vi "aaa.vi"() -> ()   [LabVIEW 2018]
uses:
  demo/Implementations/Component-A.lvclass
  U:/modules/labview-orm/_Serializable Base Object/_ISerializable.lvclass
  demo/Implementations/Product-A.lvclass
  ORM Scripter/ORM Scripter.lvclass
panel:
  out "create script 3":string
  out "create script":string
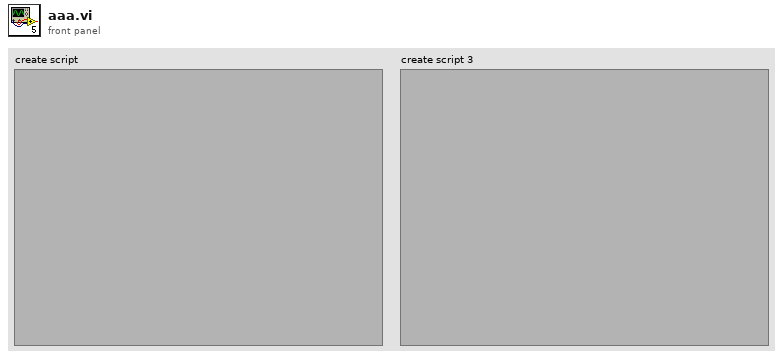
[diagram p1: front panel]
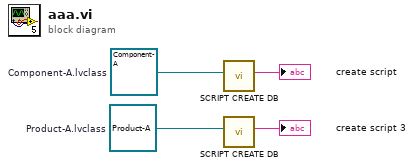
[diagram p0: block diagram]
diagram:
  w2 = refnum<class "Product-A.lvclass"> refnum  # Product-A.lvclass
  w1 = refnum<class "Component-A.lvclass"> refnum  # Component-A.lvclass
  n1 = call "SCRIPT CREATE DB.vi"("class"=w1) -> ("create script"=→"create script":string)  [unwired: 8 in, 2 out]
  n2 = call "SCRIPT CREATE DB.vi"("class"=w2) -> ("create script"=→"create script 3":string)  [unwired: 8 in, 2 out]
